vi "输入数据解析.vi"(0 "单个参数补充":dbl, 1 "从板号":dbl=1.0, 2 "主板二维码":string="BNET01", 3 "从板二维码":string="BNET01", 5 "主板引用":refnum<vi>, 7 "从板引用":refnum<vi>, 9 "主板选项":string="三级故障阀值", 11 "枚举":enum16{"主板", "从板"}(ring), 12 "快换":bool caption="快换写入") -> (4 "输出数组":dbl[][](array[numeric]), 6 "数组长度":dbl[](array[numeric]), 8 "循环次数":i32, 10 "命令":u32, 14 "名称":string[](array[string]), 15 "命令序号":u32[](array[numeric]))   [LabVIEW 2013] (continued)
                  disable-tunnel: w4127 -> [w4132 _]
                  frame Disabled {
                    n1628 = Unbundle By Name(w4132) -> ("充电电流过高"=w4131:dbl)
                    n1629 = call "输入分辨率计算-EV05.vi"("1字节?"=FALSE, "数值"=w4131, "偏移量"=-3000.0, "分辨率"=0.1) -> ("低字节"=w4133:dbl, "高字节1"=w4135:dbl)  [unwired: 1 in, 5 out]
                  }
                  frame Enabled {
                    w4138 = 255 ("高字节1")
                  }
                }
                n1630 = Build Array(w4130, w4128) -> (w4129:i32[])
              }
              frame 10 {
                # "放电电流过高"
                n1631 = disable-structure shown="启用" {
                  disable-tunnel: [w4147 w4150] -> w4142
                  disable-tunnel: [w4145 w4150] -> w4140
                  disable-tunnel: w4139 -> [w4144 _]
                  frame Disabled {
                    n1632 = Unbundle By Name(w4144) -> ("放电电流过高"=w4143:dbl)
                    n1633 = call "输入分辨率计算-EV05.vi"("1字节?"=FALSE, "数值"=w4143, "偏移量"=-3000.0, "分辨率"=0.1) -> ("低字节"=w4145:dbl, "高字节1"=w4147:dbl)  [unwired: 1 in, 5 out]
                  }
                  frame Enabled {
                    w4150 = 255 ("高字节1")
                  }
                }
                n1634 = Build Array(w4142, w4140) -> (w4141:i32[])
              }
              frame 11 {
                # "单组温度不均衡"
                n1635 = disable-structure shown="启用" {
                  disable-tunnel: [w4157 255 ("高字节1")] -> w4153
                  disable-tunnel: w4151 -> [w4155 _]
                  frame Disabled {
                    n1636 = Unbundle By Name(w4155) -> ("单组温度不均衡"=w4154:dbl)
                    n1637 = call "输入分辨率计算-EV05.vi"("1字节?"=TRUE, "数值"=w4154, "偏移量"=0.0, "分辨率"=1.0) -> ("高字节1"=w4157:dbl)  [unwired: 1 in, 6 out]
                  }
                  frame Enabled {
                  }
                }
                n1638 = Build Array(w4153) -> (w4152:i32[])
              }
              frame 12 {
                # "SOC过高"
                n1639 = Unbundle By Name(w4165) -> ("SOC过高"=w4164:dbl)
                n1640 = call "输入分辨率计算-EV05.vi"("1字节?"=FALSE, "数值"=w4164, "偏移量"=0.0, "分辨率"=0.1) -> ("低字节"=w4166:dbl, "高字节1"=w4167:dbl)  [unwired: 1 in, 5 out]
                n1641 = call "二进制解析-8.6.vi"("索引"=4, "数值"=w4167) -> ("低位子数组"=w4170:i32[])  [unwired: 3 out]
                n1642 = call "二进制解析-8.6.vi"("索引"=4, "数值"=w4166) -> ("低位子数组"=w4162:i32[], "高位子数组"=w4169:i32[])  [unwired: 2 out]
                n1643 = Insert Into Array(array=w4170, new element=w4169) -> (w4168:i32[])  [unwired: 1 in]
                n1644 = call "数值二进制转十进制-8.6.vi"("子数组"=w4168) -> ("十进制数值"=w4163:i32)  [unwired: 4 out]
                n1645 = disable-structure shown="启用" {
                  disable-tunnel: w4163 -> [w4178 _]
                  disable-tunnel: [w4178 255 ("高字节1")] -> w4161
                  disable-tunnel: [w4177 i32[] [] ("低位子数组 22")] -> _
                  disable-tunnel: w4162 -> [w4177 _]
                  frame Disabled {
                  }
                  frame Enabled {
                  }
                }
                n1646 = Build Array(w4161, w4161) -> (w4174:i32[])
              }
              frame 13 {
                # "SOC过低"
                n1647 = Unbundle By Name(w4187) -> ("SOC过低"=w4186:dbl)
                n1648 = call "输入分辨率计算-EV05.vi"("1字节?"=FALSE, "数值"=w4186, "偏移量"=0.0, "分辨率"=0.1) -> ("低字节"=w4184:dbl, "高字节1"=w4185:dbl)  [unwired: 1 in, 5 out]
                n1649 = call "二进制解析-8.6.vi"("索引"=4, "数值"=w4185) -> ("低位子数组"=w4182:i32[])  [unwired: 3 out]
                n1650 = disable-structure shown="启用" {
                  disable-tunnel: w4184 -> [w4194 _]
                  disable-tunnel: [w4194 255 ("高字节1")] -> w4183
                  disable-tunnel: w4182 -> [w4193 _]
                  disable-tunnel: [_ 255 ("高字节1")] -> w4181
                  frame Disabled {
                    (unwired) i32[] [] ("低位子数组 4")
                  }
                  frame Enabled {
                  }
                }
                n1651 = Build Array(w4181, w4183) -> (w4190:i32[])
              }
              frame 14 {
                # "内阻过大"
                n1652 = disable-structure shown="启用" {
                  disable-tunnel: w4199 -> [w4204 _]
                  disable-tunnel: [w4200 255 ("高字节1")] -> w4197
                  frame Disabled {
                    n1653 = Unbundle By Name(w4204) -> ("内阻过大"=w4203:dbl)
                    n1654 = call "输入分辨率计算-EV05.vi"("1字节?"=TRUE, "数值"=w4203, "分辨率"=0.1) -> ("高字节1"=w4200:dbl)  [unwired: 2 in, 6 out]
                  }
                  frame Enabled {
                  }
                }
                n1655 = Build Array(w4197) -> (w4198:i32[])
              }
              frame 15 {
                # "极柱温度过高"
                n1656 = disable-structure shown="启用" {
                  disable-tunnel: w4208 -> [w4214 _]
                  disable-tunnel: [w4210 255 ("高字节1")] -> w4206
                  frame Disabled {
                    n1657 = Unbundle By Name(w4214) -> ("极柱温度过高"=w4213:dbl)
                    n1658 = call "输入分辨率计算-EV05.vi"("1字节?"=TRUE, "数值"=w4213, "偏移量"=-40.0, "分辨率"=1.0) -> ("高字节1"=w4210:dbl)  [unwired: 1 in, 6 out]
                  }
                  frame Enabled {
                  }
                }
                n1659 = Build Array(w4206) -> (w4207:i32[])
              }
              frame 16 {
                # "SOH过低"
                n1660 = disable-structure shown="启用" {
                  disable-tunnel: [w4231 w4239] -> w4218
                  disable-tunnel: w4217 -> [w4228 _]
                  disable-tunnel: [w4220 w4239] -> w4216
                  frame Disabled {
                    n1661 = Unbundle By Name(w4228) -> ("SOH过低"=w4227:dbl)
                    n1662 = call "输入分辨率计算-EV05.vi"("1字节?"=FALSE, "数值"=w4227, "偏移量"=0.0, "分辨率"=0.1) -> ("低字节"=w4229:dbl, "高字节1"=w4230:dbl)  [unwired: 1 in, 5 out]
                    n1663 = call "二进制解析-8.6.vi"("索引"=4, "数值"=w4230) -> ("低位子数组"=w4233:i32[])  [unwired: 3 out]
                    n1664 = call "二进制解析-8.6.vi"("索引"=4, "数值"=w4229) -> ("低位子数组"=w4222:i32[], "高位子数组"=w4232:i32[])  [unwired: 2 out]
                    n1665 = call "二进制解析-8.6.vi"("索引"=4, "数值"=0) -> ("低位子数组"=w4223:i32[])  [unwired: 3 out]
                    n1666 = Insert Into Array(array=w4233, new element=w4232) -> (w4226:i32[])  [unwired: 1 in]
                    n1667 = Insert Into Array(array=w4222, new element=w4223) -> (w4221:i32[])  [unwired: 1 in]
                    n1668 = call "数值二进制转十进制-8.6.vi"("子数组"=w4226) -> ("十进制数值"=w4231:i32)  [unwired: 4 out]
                    n1669 = call "数值二进制转十进制-8.6.vi"("子数组"=w4221) -> ("十进制数值"=w4220:i32)  [unwired: 4 out]
                  }
                  frame Enabled {
                    w4239 = 255 ("高字节1")
                  }
                }
                n1670 = Build Array(w4218, w4216) -> (w4219:i32[])
              }
            }
            n1671 = Insert Into Array(array=w4024, new element=w4025) -> (w4023:dbl[])  [unwired: 1 in]
          }
          n1672 = Build Array(w4020) -> (w4019:dbl[][])
          n1673 = Build Array("二级故障阀值") -> (w4010:string[])
        }
        frame "整组温度不均衡(3)" {
          n1674 = Unbundle By Name(w4245) -> ("一级故障 3"=w4246:refnum<vi>)
          n1675 = property class="Clust (严格)"(reference=w4246) -> ("Value"=w4244:T4)  [unwired: 1 in, 2 out]
          n1676 = for {
            N: 17 -> [_]
            tunnel: w4244 -> [w4256]
            shift-right: [w4253] -> w4250
            shift-left: dbl[] [] -> [w4254]
            i -> [w4257]
            n1677 = case shown="4" w4257 {
              tunnel: w4256 -> [w4258 w4269 w4280 w4290 w4300 w4309 w4321 w4333 w4345 w4357 w4369 w4381 w4395 w4417 w4429 w4438 w4447]
              tunnel: [w4259 w4270 w4281 w4291 w4301 w4311 w4323 w4335 w4347 w4359 w4371 w4382 w4404 w4420 w4428 w4437 w4449] -> w4255
              frame 0, Default {
                # "总电压过高"
                n1678 = disable-structure shown="启用" {
                  disable-tunnel: [w4265 w4268] -> w4261
                  disable-tunnel: [w4264 w4268] -> w4260
                  disable-tunnel: w4258 -> [w4263 _]
                  frame Disabled {
                    n1679 = Unbundle By Name(w4263) -> ("总电压过高"=w4262:dbl)
                    n1680 = call "输入分辨率计算-EV05.vi"("1字节?"=FALSE, "数值"=w4262, "分辨率"=0.1) -> ("低字节"=w4265:dbl, "高字节1"=w4264:dbl)  [unwired: 2 in, 5 out]
                  }
                  frame Enabled {
                    w4268 = 255 ("高字节1")
                  }
                }
                n1681 = Build Array(w4260, w4261) -> (w4259:i32[])
              }
              frame 1 {
                # "总电压过低"
                n1682 = disable-structure shown="启用" {
                  disable-tunnel: [w4276 w4279] -> w4272
                  disable-tunnel: [w4275 w4279] -> w4271
                  disable-tunnel: w4269 -> [w4274 _]
                  frame Disabled {
                    n1683 = Unbundle By Name(w4274) -> ("总电压过低"=w4273:dbl)
                    n1684 = call "输入分辨率计算-EV05.vi"("1字节?"=FALSE, "数值"=w4273, "分辨率"=0.1) -> ("低字节"=w4276:dbl, "高字节1"=w4275:dbl)  [unwired: 2 in, 5 out]
                  }
                  frame Enabled {
                    w4279 = 255 ("高字节1")
                  }
                }
                n1685 = Build Array(w4271, w4272) -> (w4270:i32[])
              }
              frame 2 {
                # "温度过高"
                n1686 = disable-structure shown="启用" {
                  disable-tunnel: [w4286 255 ("高字节1")] -> w4282
                  disable-tunnel: w4280 -> [w4284 _]
                  frame Disabled {
                    n1687 = Unbundle By Name(w4284) -> ("温度过高"=w4283:dbl)
                    n1688 = call "输入分辨率计算-EV05.vi"("1字节?"=TRUE, "数值"=w4283, "偏移量"=-40.0, "分辨率"=1.0) -> ("高字节1"=w4286:dbl)  [unwired: 1 in, 6 out]
                  }
                  frame Enabled {
                  }
                }
                n1689 = Build Array(w4282) -> (w4281:i32[])
              }
              frame 3 {
                # "温度过低"
                n1690 = disable-structure shown="启用" {
                  disable-tunnel: [w4296 255 ("高字节1")] -> w4292
                  disable-tunnel: w4290 -> [w4294 _]
                  frame Disabled {
                    n1691 = Unbundle By Name(w4294) -> ("温度过低"=w4293:dbl)
                    n1692 = call "输入分辨率计算-EV05.vi"("1字节?"=TRUE, "数值"=w4293, "偏移量"=-40.0, "分辨率"=1.0) -> ("高字节1"=w4296:dbl)  [unwired: 1 in, 6 out]
                  }
                  frame Enabled {
                  }
                }
                n1693 = Build Array(w4292) -> (w4291:i32[])
              }
              frame 4 {
                # "整组温度不均衡"
                n1694 = disable-structure shown="启用" {
                  disable-tunnel: [w4305 255 ("高字节1")] -> w4302
                  disable-tunnel: w4300 -> [w4304 _]
                  frame Enabled {
                    n1695 = Unbundle By Name(w4304) -> ("整组温度不均衡"=w4303:dbl)
                    n1696 = call "输入分辨率计算-EV05.vi"("1字节?"=TRUE, "数值"=w4303, "分辨率"=1.0) -> ("高字节1"=w4305:dbl)  [unwired: 2 in, 6 out]
                  }
                  frame Disabled {
                  }
                }
                n1697 = Build Array(w4302) -> (w4301:dbl[])
              }
              frame 5 {
                # "单组电压不均衡"
                n1698 = disable-structure shown="启用" {
                  disable-tunnel: [w4317 w4320] -> w4312
                  disable-tunnel: [w4315 w4320] -> w4310
                  disable-tunnel: w4309 -> [w4314 _]
                  frame Disabled {
                    n1699 = Unbundle By Name(w4314) -> ("单组电压不均衡"=w4313:dbl)
                    n1700 = call "输入分辨率计算-EV05.vi"("1字节?"=FALSE, "数值"=w4313, "偏移量"=0.0, "分辨率"=0.001) -> ("低字节"=w4315:dbl, "高字节1"=w4317:dbl)  [unwired: 1 in, 5 out]
                  }
                  frame Enabled {
                    w4320 = 255 ("高字节1")
                  }
                }
                n1701 = Build Array(w4312, w4310) -> (w4311:i32[])
              }
              frame 6 {
                # "整组电压不均衡"
                n1702 = disable-structure shown="启用" {
                  disable-tunnel: [w4329 w4332] -> w4324
                  disable-tunnel: [w4327 w4332] -> w4322
                  disable-tunnel: w4321 -> [w4326 _]
                  frame Disabled {
                    n1703 = Unbundle By Name(w4326) -> ("整组电压不均衡"=w4325:dbl)
                    n1704 = call "输入分辨率计算-EV05.vi"("1字节?"=FALSE, "数值"=w4325, "偏移量"=0.0, "分辨率"=0.001) -> ("低字节"=w4327:dbl, "高字节1"=w4329:dbl)  [unwired: 1 in, 5 out]
                  }
                  frame Enabled {
                    w4332 = 255 ("高字节1")
                  }
                }
                n1705 = Build Array(w4324, w4322) -> (w4323:i32[])
              }
              frame 7 {
                # "单体电压过高"
                n1706 = disable-structure shown="启用" {
                  disable-tunnel: [w4341 w4344] -> w4336
                  disable-tunnel: [w4339 w4344] -> w4334
                  disable-tunnel: w4333 -> [w4338 _]
                  frame Disabled {
                    n1707 = Unbundle By Name(w4338) -> ("单体电压过高"=w4337:dbl)
                    n1708 = call "输入分辨率计算-EV05.vi"("1字节?"=FALSE, "数值"=w4337, "偏移量"=0.0, "分辨率"=0.001) -> ("低字节"=w4339:dbl, "高字节1"=w4341:dbl)  [unwired: 1 in, 5 out]
                  }
                  frame Enabled {
                    w4344 = 255 ("高字节1")
                  }
                }
                n1709 = Build Array(w4336, w4334) -> (w4335:i32[])
              }
              frame 8 {
                # "单体电压过低"
                n1710 = disable-structure shown="启用" {
                  disable-tunnel: [w4353 w4356] -> w4348
                  disable-tunnel: [w4351 w4356] -> w4346
                  disable-tunnel: w4345 -> [w4350 _]
                  frame Disabled {
                    n1711 = Unbundle By Name(w4350) -> ("单体电压过低"=w4349:dbl)
                    n1712 = call "输入分辨率计算-EV05.vi"("1字节?"=FALSE, "数值"=w4349, "偏移量"=0.0, "分辨率"=0.001) -> ("低字节"=w4351:dbl, "高字节1"=w4353:dbl)  [unwired: 1 in, 5 out]
                  }
                  frame Enabled {
                    w4356 = 255 ("高字节1")
                  }
                }
                n1713 = Build Array(w4348, w4346) -> (w4347:i32[])
              }
              frame 9 {
                # "充电电流过高"
                n1714 = disable-structure shown="启用" {
                  disable-tunnel: [w4365 w4368] -> w4360
                  disable-tunnel: [w4363 w4368] -> w4358
                  disable-tunnel: w4357 -> [w4362 _]
                  frame Disabled {
                    n1715 = Unbundle By Name(w4362) -> ("充电电流过高"=w4361:dbl)
                    n1716 = call "输入分辨率计算-EV05.vi"("1字节?"=FALSE, "数值"=w4361, "偏移量"=-3000.0, "分辨率"=0.1) -> ("低字节"=w4363:dbl, "高字节1"=w4365:dbl)  [unwired: 1 in, 5 out]
                  }
                  frame Enabled {
                    w4368 = 255 ("高字节1")
                  }
                }
                n1717 = Build Array(w4360, w4358) -> (w4359:i32[])
              }
              frame 10 {
                # "放电电流过高"
                n1718 = disable-structure shown="启用" {
                  disable-tunnel: [w4377 w4380] -> w4372
                  disable-tunnel: [w4375 w4380] -> w4370
                  disable-tunnel: w4369 -> [w4374 _]
                  frame Disabled {
                    n1719 = Unbundle By Name(w4374) -> ("放电电流过高"=w4373:dbl)
                    n1720 = call "输入分辨率计算-EV05.vi"("1字节?"=FALSE, "数值"=w4373, "偏移量"=-3000.0, "分辨率"=0.1) -> ("低字节"=w4375:dbl, "高字节1"=w4377:dbl)  [unwired: 1 in, 5 out]
                  }
                  frame Enabled {
                    w4380 = 255 ("高字节1")
                  }
                }
                n1721 = Build Array(w4372, w4370) -> (w4371:i32[])
              }
              frame 11 {
                # "单组温度不均衡"
                n1722 = disable-structure shown="启用" {
                  disable-tunnel: [w4387 255 ("高字节1")] -> w4383
                  disable-tunnel: w4381 -> [w4385 _]
                  frame Disabled {
                    n1723 = Unbundle By Name(w4385) -> ("单组温度不均衡"=w4384:dbl)
                    n1724 = call "输入分辨率计算-EV05.vi"("1字节?"=TRUE, "数值"=w4384, "偏移量"=0.0, "分辨率"=1.0) -> ("高字节1"=w4387:dbl)  [unwired: 1 in, 6 out]
                  }
                  frame Enabled {
                  }
                }
                n1725 = Build Array(w4383) -> (w4382:i32[])
              }
              frame 12 {
                # "SOC过高"
                n1726 = Unbundle By Name(w4395) -> ("SOC过高"=w4394:dbl)
                n1727 = call "输入分辨率计算-EV05.vi"("1字节?"=FALSE, "数值"=w4394, "偏移量"=0.0, "分辨率"=0.1) -> ("低字节"=w4396:dbl, "高字节1"=w4397:dbl)  [unwired: 1 in, 5 out]
                n1728 = call "二进制解析-8.6.vi"("索引"=4, "数值"=w4397) -> ("低位子数组"=w4400:i32[])  [unwired: 3 out]
                n1729 = call "二进制解析-8.6.vi"("索引"=4, "数值"=w4396) -> ("低位子数组"=w4392:i32[], "高位子数组"=w4399:i32[])  [unwired: 2 out]
                n1730 = Insert Into Array(array=w4400, new element=w4399) -> (w4398:i32[])  [unwired: 1 in]
                n1731 = call "数值二进制转十进制-8.6.vi"("子数组"=w4398) -> ("十进制数值"=w4393:i32)  [unwired: 4 out]
                n1732 = disable-structure shown="启用" {
                  disable-tunnel: w4393 -> [w4408 _]
                  disable-tunnel: [w4408 255 ("高字节1")] -> w4391
                  disable-tunnel: [w4407 i32[] [] ("低位子数组 22")] -> _
                  disable-tunnel: w4392 -> [w4407 _]
                  frame Disabled {
                  }
                  frame Enabled {
                  }
                }
                n1733 = Build Array(w4391, w4391) -> (w4404:i32[])
              }
              frame 13 {
                # "SOC过低"
                n1734 = Unbundle By Name(w4417) -> ("SOC过低"=w4416:dbl)
                n1735 = call "输入分辨率计算-EV05.vi"("1字节?"=FALSE, "数值"=w4416, "偏移量"=0.0, "分辨率"=0.1) -> ("低字节"=w4414:dbl, "高字节1"=w4415:dbl)  [unwired: 1 in, 5 out]
                n1736 = call "二进制解析-8.6.vi"("索引"=4, "数值"=w4415) -> ("低位子数组"=w4412:i32[])  [unwired: 3 out]
                n1737 = disable-structure shown="启用" {
                  disable-tunnel: w4414 -> [w4424 _]
                  disable-tunnel: [w4424 255 ("高字节1")] -> w4413
                  disable-tunnel: w4412 -> [w4423 _]
                  disable-tunnel: [_ 255 ("高字节1")] -> w4411
                  frame Disabled {
                    (unwired) i32[] [] ("低位子数组 4")
                  }
                  frame Enabled {
                  }
                }
                n1738 = Build Array(w4411, w4413) -> (w4420:i32[])
              }
              frame 14 {
                # "内阻过大"
                n1739 = disable-structure shown="启用" {
                  disable-tunnel: w4429 -> [w4434 _]
                  disable-tunnel: [w4430 255 ("高字节1")] -> w4427
                  frame Disabled {
                    n1740 = Unbundle By Name(w4434) -> ("内阻过大"=w4433:dbl)
                    n1741 = call "输入分辨率计算-EV05.vi"("1字节?"=TRUE, "数值"=w4433, "分辨率"=0.1) -> ("高字节1"=w4430:dbl)  [unwired: 2 in, 6 out]
                  }
                  frame Enabled {
                  }
                }
                n1742 = Build Array(w4427) -> (w4428:i32[])
              }
              frame 15 {
                # "极柱温度过高"
                n1743 = disable-structure shown="启用" {
                  disable-tunnel: w4438 -> [w4444 _]
                  disable-tunnel: [w4440 255 ("高字节1")] -> w4436
                  frame Disabled {
                    n1744 = Unbundle By Name(w4444) -> ("极柱温度过高"=w4443:dbl)
                    n1745 = call "输入分辨率计算-EV05.vi"("1字节?"=TRUE, "数值"=w4443, "偏移量"=-40.0, "分辨率"=1.0) -> ("高字节1"=w4440:dbl)  [unwired: 1 in, 6 out]
                  }
                  frame Enabled {
                  }
                }
                n1746 = Build Array(w4436) -> (w4437:i32[])
              }
              frame 16 {
                # "SOH过低"
                n1747 = disable-structure shown="启用" {
                  disable-tunnel: [w4461 w4469] -> w4448
                  disable-tunnel: w4447 -> [w4458 _]
                  disable-tunnel: [w4450 w4469] -> w4446
                  frame Disabled {
                    n1748 = Unbundle By Name(w4458) -> ("SOH过低"=w4457:dbl)
                    n1749 = call "输入分辨率计算-EV05.vi"("1字节?"=FALSE, "数值"=w4457, "偏移量"=0.0, "分辨率"=0.1) -> ("低字节"=w4459:dbl, "高字节1"=w4460:dbl)  [unwired: 1 in, 5 out]
                    n1750 = call "二进制解析-8.6.vi"("索引"=4, "数值"=w4460) -> ("低位子数组"=w4463:i32[])  [unwired: 3 out]
                    n1751 = call "二进制解析-8.6.vi"("索引"=4, "数值"=w4459) -> ("低位子数组"=w4452:i32[], "高位子数组"=w4462:i32[])  [unwired: 2 out]
                    n1752 = call "二进制解析-8.6.vi"("索引"=4, "数值"=0) -> ("低位子数组"=w4453:i32[])  [unwired: 3 out]
                    n1753 = Insert Into Array(array=w4463, new element=w4462) -> (w4456:i32[])  [unwired: 1 in]
                    n1754 = Insert Into Array(array=w4452, new element=w4453) -> (w4451:i32[])  [unwired: 1 in]
                    n1755 = call "数值二进制转十进制-8.6.vi"("子数组"=w4456) -> ("十进制数值"=w4461:i32)  [unwired: 4 out]
                    n1756 = call "数值二进制转十进制-8.6.vi"("子数组"=w4451) -> ("十进制数值"=w4450:i32)  [unwired: 4 out]
                  }
                  frame Enabled {
                    w4469 = 255 ("高字节1")
                  }
                }
                n1757 = Build Array(w4448, w4446) -> (w4449:i32[])
              }
            }
            n1758 = Insert Into Array(array=w4254, new element=w4255) -> (w4253:dbl[])  [unwired: 1 in]
          }
          n1759 = Build Array(w4250) -> (w4249:dbl[][])
          n1760 = Build Array("三级故障阀值") -> (w4240:string[])
        }
        frame "单组电压不均衡" {
          n1761 = Unbundle By Name(w4475) -> ("一级故障"=w4476:refnum<vi>)
          n1762 = property class="Clust (严格)"(reference=w4476) -> ("Value"=w4474:T4)  [unwired: 1 in, 2 out]
          n1763 = for {
            N: 17 -> [_]
            tunnel: w4474 -> [w4486]
            shift-right: [w4483] -> w4480
            shift-left: dbl[] [] -> [w4484]
            i -> [w4487]
            n1764 = case shown="13" w4487 {
              tunnel: w4486 -> [w4488 w4499 w4510 w4520 w4530 w4540 w4552 w4564 w4576 w4588 w4600 w4612 w4626 w4648 w4660 w4669 w4678]
              tunnel: [w4489 w4500 w4511 w4521 w4531 w4542 w4554 w4566 w4578 w4590 w4602 w4613 w4635 w4651 w4659 w4668 w4680] -> w4485
              frame 0, Default {
                # "总电压过高"
                n1765 = disable-structure shown="启用" {
                  disable-tunnel: [w4495 w4498] -> w4491
                  disable-tunnel: [w4494 w4498] -> w4490
                  disable-tunnel: w4488 -> [w4493 _]
                  frame Disabled {
                    n1766 = Unbundle By Name(w4493) -> ("总电压过高"=w4492:dbl)
                    n1767 = call "输入分辨率计算-EV05.vi"("1字节?"=FALSE, "数值"=w4492, "分辨率"=0.1) -> ("低字节"=w4495:dbl, "高字节1"=w4494:dbl)  [unwired: 2 in, 5 out]
                  }
                  frame Enabled {
                    w4498 = 255 ("高字节1")
                  }
                }
                n1768 = Build Array(w4490, w4491) -> (w4489:i32[])
              }
              frame 1 {
                # "总电压过低"
                n1769 = disable-structure shown="启用" {
                  disable-tunnel: [w4506 w4509] -> w4502
                  disable-tunnel: [w4505 w4509] -> w4501
                  disable-tunnel: w4499 -> [w4504 _]
                  frame Disabled {
                    n1770 = Unbundle By Name(w4504) -> ("总电压过低"=w4503:dbl)
                    n1771 = call "输入分辨率计算-EV05.vi"("1字节?"=FALSE, "数值"=w4503, "分辨率"=0.1) -> ("低字节"=w4506:dbl, "高字节1"=w4505:dbl)  [unwired: 2 in, 5 out]
                  }
                  frame Enabled {
                    w4509 = 255 ("高字节1")
                  }
                }
                n1772 = Build Array(w4501, w4502) -> (w4500:i32[])
              }
              frame 2 {
                # "温度过高"
                n1773 = disable-structure shown="启用" {
                  disable-tunnel: [w4516 255 ("高字节1")] -> w4512
                  disable-tunnel: w4510 -> [w4514 _]
                  frame Disabled {
                    n1774 = Unbundle By Name(w4514) -> ("温度过高"=w4513:dbl)
                    n1775 = call "输入分辨率计算-EV05.vi"("1字节?"=TRUE, "数值"=w4513, "偏移量"=-40.0, "分辨率"=1.0) -> ("高字节1"=w4516:dbl)  [unwired: 1 in, 6 out]
                  }
                  frame Enabled {
                  }
                }
                n1776 = Build Array(w4512) -> (w4511:i32[])
              }
              frame 3 {
                # "温度过低"
                n1777 = disable-structure shown="启用" {
                  disable-tunnel: [w4526 255 ("高字节1")] -> w4522
                  disable-tunnel: w4520 -> [w4524 _]
                  frame Disabled {
                    n1778 = Unbundle By Name(w4524) -> ("温度过低"=w4523:dbl)
                    n1779 = call "输入分辨率计算-EV05.vi"("1字节?"=TRUE, "数值"=w4523, "偏移量"=-40.0, "分辨率"=1.0) -> ("高字节1"=w4526:dbl)  [unwired: 1 in, 6 out]
                  }
                  frame Enabled {
                  }
                }
                n1780 = Build Array(w4522) -> (w4521:i32[])
              }
              frame 4 {
                # "整组温度不均衡"
                n1781 = disable-structure shown="启用" {
                  disable-tunnel: [w4536 255 ("高字节1")] -> w4532
                  disable-tunnel: w4530 -> [w4534 _]
                  frame Disabled {
                    n1782 = Unbundle By Name(w4534) -> ("整组温度不均衡"=w4533:dbl)
                    n1783 = call "输入分辨率计算-EV05.vi"("1字节?"=TRUE, "数值"=w4533, "偏移量"=0.0, "分辨率"=1.0) -> ("高字节1"=w4536:dbl)  [unwired: 1 in, 6 out]
                  }
                  frame Enabled {
                  }
                }
                n1784 = Build Array(w4532) -> (w4531:i32[])
              }
              frame 5 {
                # "单组电压不均衡"
                n1785 = disable-structure shown="启用" {
                  disable-tunnel: [w4548 w4551] -> w4543
                  disable-tunnel: [w4546 w4551] -> w4541
                  disable-tunnel: w4540 -> [w4545 _]
                  frame Enabled {
                    n1786 = Unbundle By Name(w4545) -> ("单组电压不均衡"=w4544:dbl)
                    n1787 = call "输入分辨率计算-EV05.vi"("1字节?"=FALSE, "数值"=w4544, "偏移量"=0.0, "分辨率"=0.001) -> ("低字节"=w4546:dbl, "高字节1"=w4548:dbl)  [unwired: 1 in, 5 out]
                  }
                  frame Disabled {
                    w4551 = 255 ("高字节1")
                  }
                }
                n1788 = Build Array(w4543, w4541) -> (w4542:dbl[])
              }
              frame 6 {
                # "整组电压不均衡"
                n1789 = disable-structure shown="启用" {
                  disable-tunnel: [w4560 w4563] -> w4555
                  disable-tunnel: [w4558 w4563] -> w4553
                  disable-tunnel: w4552 -> [w4557 _]
                  frame Disabled {
                    n1790 = Unbundle By Name(w4557) -> ("整组电压不均衡"=w4556:dbl)
                    n1791 = call "输入分辨率计算-EV05.vi"("1字节?"=FALSE, "数值"=w4556, "偏移量"=0.0, "分辨率"=0.001) -> ("低字节"=w4558:dbl, "高字节1"=w4560:dbl)  [unwired: 1 in, 5 out]
                  }
                  frame Enabled {
                    w4563 = 255 ("高字节1")
                  }
                }
                n1792 = Build Array(w4555, w4553) -> (w4554:i32[])
              }
              frame 7 {
                # "单体电压过高"
                n1793 = disable-structure shown="启用" {
                  disable-tunnel: [w4572 w4575] -> w4567
                  disable-tunnel: [w4570 w4575] -> w4565
                  disable-tunnel: w4564 -> [w4569 _]
                  frame Disabled {
                    n1794 = Unbundle By Name(w4569) -> ("单体电压过高"=w4568:dbl)
                    n1795 = call "输入分辨率计算-EV05.vi"("1字节?"=FALSE, "数值"=w4568, "偏移量"=0.0, "分辨率"=0.001) -> ("低字节"=w4570:dbl, "高字节1"=w4572:dbl)  [unwired: 1 in, 5 out]
                  }
                  frame Enabled {
                    w4575 = 255 ("高字节1")
                  }
                }
                n1796 = Build Array(w4567, w4565) -> (w4566:i32[])
              }
              frame 8 {
                # "单体电压过低"
                n1797 = disable-structure shown="启用" {
                  disable-tunnel: [w4584 w4587] -> w4579
                  disable-tunnel: [w4582 w4587] -> w4577
                  disable-tunnel: w4576 -> [w4581 _]
                  frame Disabled {
                    n1798 = Unbundle By Name(w4581) -> ("单体电压过低"=w4580:dbl)
                    n1799 = call "输入分辨率计算-EV05.vi"("1字节?"=FALSE, "数值"=w4580, "偏移量"=0.0, "分辨率"=0.001) -> ("低字节"=w4582:dbl, "高字节1"=w4584:dbl)  [unwired: 1 in, 5 out]
                  }
                  frame Enabled {
                    w4587 = 255 ("高字节1")
                  }
                }
                n1800 = Build Array(w4579, w4577) -> (w4578:i32[])
              }
              frame 9 {
                # "充电电流过高"
                n1801 = disable-structure shown="启用" {
                  disable-tunnel: [w4596 w4599] -> w4591
                  disable-tunnel: [w4594 w4599] -> w4589
                  disable-tunnel: w4588 -> [w4593 _]
                  frame Disabled {
                    n1802 = Unbundle By Name(w4593) -> ("充电电流过高"=w4592:dbl)
                    n1803 = call "输入分辨率计算-EV05.vi"("1字节?"=FALSE, "数值"=w4592, "偏移量"=-3000.0, "分辨率"=0.1) -> ("低字节"=w4594:dbl, "高字节1"=w4596:dbl)  [unwired: 1 in, 5 out]
                  }
                  frame Enabled {
                    w4599 = 255 ("高字节1")
                  }
                }
                n1804 = Build Array(w4591, w4589) -> (w4590:i32[])
              }
              frame 10 {
                # "放电电流过高"
                n1805 = disable-structure shown="启用" {
                  disable-tunnel: [w4608 w4611] -> w4603
                  disable-tunnel: [w4606 w4611] -> w4601
                  disable-tunnel: w4600 -> [w4605 _]
                  frame Disabled {
                    n1806 = Unbundle By Name(w4605) -> ("放电电流过高"=w4604:dbl)
                    n1807 = call "输入分辨率计算-EV05.vi"("1字节?"=FALSE, "数值"=w4604, "偏移量"=-3000.0, "分辨率"=0.1) -> ("低字节"=w4606:dbl, "高字节1"=w4608:dbl)  [unwired: 1 in, 5 out]
                  }
                  frame Enabled {
                    w4611 = 255 ("高字节1")
                  }
                }
                n1808 = Build Array(w4603, w4601) -> (w4602:i32[])
              }
              frame 11 {
                # "单组温度不均衡"
                n1809 = disable-structure shown="启用" {
                  disable-tunnel: [w4618 255 ("高字节1")] -> w4614
                  disable-tunnel: w4612 -> [w4616 _]
                  frame Disabled {
                    n1810 = Unbundle By Name(w4616) -> ("单组温度不均衡"=w4615:dbl)
                    n1811 = call "输入分辨率计算-EV05.vi"("1字节?"=TRUE, "数值"=w4615, "偏移量"=0.0, "分辨率"=1.0) -> ("高字节1"=w4618:dbl)  [unwired: 1 in, 6 out]
                  }
                  frame Enabled {
                  }
                }
                n1812 = Build Array(w4614) -> (w4613:i32[])
              }
              frame 12 {
                # "SOC过高"
                n1813 = Unbundle By Name(w4626) -> ("SOC过高"=w4625:dbl)
                n1814 = call "输入分辨率计算-EV05.vi"("1字节?"=FALSE, "数值"=w4625, "偏移量"=0.0, "分辨率"=0.1) -> ("低字节"=w4627:dbl, "高字节1"=w4628:dbl)  [unwired: 1 in, 5 out]
                n1815 = call "二进制解析-8.6.vi"("索引"=4, "数值"=w4628) -> ("低位子数组"=w4631:i32[])  [unwired: 3 out]
                n1816 = call "二进制解析-8.6.vi"("索引"=4, "数值"=w4627) -> ("低位子数组"=w4623:i32[], "高位子数组"=w4630:i32[])  [unwired: 2 out]
                n1817 = Insert Into Array(array=w4631, new element=w4630) -> (w4629:i32[])  [unwired: 1 in]
                n1818 = call "数值二进制转十进制-8.6.vi"("子数组"=w4629) -> ("十进制数值"=w4624:i32)  [unwired: 4 out]
                n1819 = disable-structure shown="启用" {
                  disable-tunnel: w4624 -> [w4639 _]
                  disable-tunnel: [w4639 255 ("高字节1")] -> w4622
                  disable-tunnel: [w4638 i32[] [] ("低位子数组 23")] -> _
                  disable-tunnel: w4623 -> [w4638 _]
                  frame Disabled {
                  }
                  frame Enabled {
                  }
                }
                n1820 = Build Array(w4622, w4622) -> (w4635:i32[])
              }
              frame 13 {
                # "SOC过低"
                n1821 = Unbundle By Name(w4648) -> ("SOC过低"=w4647:dbl)
                n1822 = call "输入分辨率计算-EV05.vi"("1字节?"=FALSE, "数值"=w4647, "偏移量"=0.0, "分辨率"=0.1) -> ("低字节"=w4645:dbl, "高字节1"=w4646:dbl)  [unwired: 1 in, 5 out]
                n1823 = call "二进制解析-8.6.vi"("索引"=4, "数值"=w4646) -> ("低位子数组"=w4643:i32[])  [unwired: 3 out]
                n1824 = disable-structure shown="启用" {
                  disable-tunnel: w4645 -> [w4655 _]
                  disable-tunnel: [w4655 255 ("高字节1")] -> w4644
                  disable-tunnel: w4643 -> [w4654 _]
                  disable-tunnel: [_ 255 ("高字节1")] -> w4642
                  frame Disabled {
                    (unwired) i32[] [] ("低位子数组 4")
                  }
                  frame Enabled {
                  }
                }
                n1825 = Build Array(w4642, w4644) -> (w4651:i32[])
              }
              frame 14 {
                # "内阻过大"
                n1826 = disable-structure shown="启用" {
                  disable-tunnel: w4660 -> [w4665 _]
                  disable-tunnel: [w4661 255 ("高字节1")] -> w4658
                  frame Disabled {
                    n1827 = Unbundle By Name(w4665) -> ("内阻过大"=w4664:dbl)
                    n1828 = call "输入分辨率计算-EV05.vi"("1字节?"=TRUE, "数值"=w4664, "分辨率"=0.1) -> ("高字节1"=w4661:dbl)  [unwired: 2 in, 6 out]
                  }
                  frame Enabled {
                  }
                }
                n1829 = Build Array(w4658) -> (w4659:i32[])
              }
              frame 15 {
                # "极柱温度过高"
                n1830 = disable-structure shown="启用" {
                  disable-tunnel: w4669 -> [w4675 _]
                  disable-tunnel: [w4671 255 ("高字节1")] -> w4667
                  frame Disabled {
                    n1831 = Unbundle By Name(w4675) -> ("极柱温度过高"=w4674:dbl)
                    n1832 = call "输入分辨率计算-EV05.vi"("1字节?"=TRUE, "数值"=w4674, "偏移量"=-40.0, "分辨率"=1.0) -> ("高字节1"=w4671:dbl)  [unwired: 1 in, 6 out]
                  }
                  frame Enabled {
                  }
                }
                n1833 = Build Array(w4667) -> (w4668:i32[])
              }
              frame 16 {
                # "SOH过低"
                n1834 = disable-structure shown="启用" {
                  disable-tunnel: [w4692 w4700] -> w4679
                  disable-tunnel: w4678 -> [w4689 _]
                  disable-tunnel: [w4681 w4700] -> w4677
                  frame Disabled {
                    n1835 = Unbundle By Name(w4689) -> ("SOH过低"=w4688:dbl)
                    n1836 = call "输入分辨率计算-EV05.vi"("1字节?"=FALSE, "数值"=w4688, "偏移量"=0.0, "分辨率"=0.1) -> ("低字节"=w4690:dbl, "高字节1"=w4691:dbl)  [unwired: 1 in, 5 out]
                    n1837 = call "二进制解析-8.6.vi"("索引"=4, "数值"=w4691) -> ("低位子数组"=w4694:i32[])  [unwired: 3 out]
                    n1838 = call "二进制解析-8.6.vi"("索引"=4, "数值"=w4690) -> ("低位子数组"=w4683:i32[], "高位子数组"=w4693:i32[])  [unwired: 2 out]
                    n1839 = call "二进制解析-8.6.vi"("索引"=4, "数值"=0) -> ("低位子数组"=w4684:i32[])  [unwired: 3 out]
                    n1840 = Insert Into Array(array=w4694, new element=w4693) -> (w4687:i32[])  [unwired: 1 in]
                    n1841 = Insert Into Array(array=w4683, new element=w4684) -> (w4682:i32[])  [unwired: 1 in]
                    n1842 = call "数值二进制转十进制-8.6.vi"("子数组"=w4687) -> ("十进制数值"=w4692:i32)  [unwired: 4 out]
                    n1843 = call "数值二进制转十进制-8.6.vi"("子数组"=w4682) -> ("十进制数值"=w4681:i32)  [unwired: 4 out]
                  }
                  frame Enabled {
                    w4700 = 255 ("高字节1")
                  }
                }
                n1844 = Build Array(w4679, w4677) -> (w4680:i32[])
              }
            }
            n1845 = Insert Into Array(array=w4484, new element=w4485) -> (w4483:dbl[])  [unwired: 1 in]
          }
          n1846 = Build Array(w4480) -> (w4479:dbl[][])
          n1847 = Build Array("一级故障阀值") -> (w4470:string[])
        }
        frame "单组电压不均衡(2)" {
          n1848 = Unbundle By Name(w4706) -> ("一级故障 2"=w4707:refnum<vi>)
          n1849 = property class="Clust (严格)"(reference=w4707) -> ("Value"=w4705:T4)  [unwired: 1 in, 2 out]
          n1850 = for {
            N: 17 -> [_]
            tunnel: w4705 -> [w4717]
            shift-right: [w4714] -> w4711
            shift-left: dbl[] [] -> [w4715]
            i -> [w4718]
            n1851 = case shown="13" w4718 {
              tunnel: w4717 -> [w4719 w4730 w4741 w4751 w4761 w4771 w4783 w4795 w4807 w4819 w4831 w4843 w4857 w4879 w4891 w4900 w4909]
              tunnel: [w4720 w4731 w4742 w4752 w4762 w4773 w4785 w4797 w4809 w4821 w4833 w4844 w4866 w4882 w4890 w4899 w4911] -> w4716
              frame 0, Default {
                # "总电压过高"
                n1852 = disable-structure shown="启用" {
                  disable-tunnel: [w4726 w4729] -> w4722
                  disable-tunnel: [w4725 w4729] -> w4721
                  disable-tunnel: w4719 -> [w4724 _]
                  frame Disabled {
                    n1853 = Unbundle By Name(w4724) -> ("总电压过高"=w4723:dbl)
                    n1854 = call "输入分辨率计算-EV05.vi"("1字节?"=FALSE, "数值"=w4723, "分辨率"=0.1) -> ("低字节"=w4726:dbl, "高字节1"=w4725:dbl)  [unwired: 2 in, 5 out]
                  }
                  frame Enabled {
                    w4729 = 255 ("高字节1")
                  }
                }
                n1855 = Build Array(w4721, w4722) -> (w4720:i32[])
              }
              frame 1 {
                # "总电压过低"
                n1856 = disable-structure shown="启用" {
                  disable-tunnel: [w4737 w4740] -> w4733
                  disable-tunnel: [w4736 w4740] -> w4732
                  disable-tunnel: w4730 -> [w4735 _]
                  frame Disabled {
                    n1857 = Unbundle By Name(w4735) -> ("总电压过低"=w4734:dbl)
                    n1858 = call "输入分辨率计算-EV05.vi"("1字节?"=FALSE, "数值"=w4734, "分辨率"=0.1) -> ("低字节"=w4737:dbl, "高字节1"=w4736:dbl)  [unwired: 2 in, 5 out]
                  }
                  frame Enabled {
                    w4740 = 255 ("高字节1")
                  }
                }
                n1859 = Build Array(w4732, w4733) -> (w4731:i32[])
              }
              frame 2 {
                # "温度过高"
                n1860 = disable-structure shown="启用" {
                  disable-tunnel: [w4747 255 ("高字节1")] -> w4743
                  disable-tunnel: w4741 -> [w4745 _]
                  frame Disabled {
                    n1861 = Unbundle By Name(w4745) -> ("温度过高"=w4744:dbl)
                    n1862 = call "输入分辨率计算-EV05.vi"("1字节?"=TRUE, "数值"=w4744, "偏移量"=-40.0, "分辨率"=1.0) -> ("高字节1"=w4747:dbl)  [unwired: 1 in, 6 out]
                  }
                  frame Enabled {
                  }
                }
                n1863 = Build Array(w4743) -> (w4742:i32[])
              }
              frame 3 {
                # "温度过低"
                n1864 = disable-structure shown="启用" {
                  disable-tunnel: [w4757 255 ("高字节1")] -> w4753
                  disable-tunnel: w4751 -> [w4755 _]
                  frame Disabled {
                    n1865 = Unbundle By Name(w4755) -> ("温度过低"=w4754:dbl)
                    n1866 = call "输入分辨率计算-EV05.vi"("1字节?"=TRUE, "数值"=w4754, "偏移量"=-40.0, "分辨率"=1.0) -> ("高字节1"=w4757:dbl)  [unwired: 1 in, 6 out]
                  }
                  frame Enabled {
                  }
                }
                n1867 = Build Array(w4753) -> (w4752:i32[])
              }
              frame 4 {
                # "整组温度不均衡"
                n1868 = disable-structure shown="启用" {
                  disable-tunnel: [w4767 255 ("高字节1")] -> w4763
                  disable-tunnel: w4761 -> [w4765 _]
                  frame Disabled {
                    n1869 = Unbundle By Name(w4765) -> ("整组温度不均衡"=w4764:dbl)
                    n1870 = call "输入分辨率计算-EV05.vi"("1字节?"=TRUE, "数值"=w4764, "偏移量"=0.0, "分辨率"=1.0) -> ("高字节1"=w4767:dbl)  [unwired: 1 in, 6 out]
                  }
                  frame Enabled {
                  }
                }
                n1871 = Build Array(w4763) -> (w4762:i32[])
              }
              frame 5 {
                # "单组电压不均衡"
                n1872 = disable-structure shown="启用" {
                  disable-tunnel: [w4779 w4782] -> w4774
                  disable-tunnel: [w4777 w4782] -> w4772
                  disable-tunnel: w4771 -> [w4776 _]
                  frame Enabled {
                    n1873 = Unbundle By Name(w4776) -> ("单组电压不均衡"=w4775:dbl)
                    n1874 = call "输入分辨率计算-EV05.vi"("1字节?"=FALSE, "数值"=w4775, "偏移量"=0.0, "分辨率"=0.001) -> ("低字节"=w4777:dbl, "高字节1"=w4779:dbl)  [unwired: 1 in, 5 out]
                  }
                  frame Disabled {
                    w4782 = 255 ("高字节1")
                  }
                }
                n1875 = Build Array(w4774, w4772) -> (w4773:dbl[])
              }
              frame 6 {
                # "整组电压不均衡"
                n1876 = disable-structure shown="启用" {
                  disable-tunnel: [w4791 w4794] -> w4786
                  disable-tunnel: [w4789 w4794] -> w4784
                  disable-tunnel: w4783 -> [w4788 _]
                  frame Disabled {
                    n1877 = Unbundle By Name(w4788) -> ("整组电压不均衡"=w4787:dbl)
                    n1878 = call "输入分辨率计算-EV05.vi"("1字节?"=FALSE, "数值"=w4787, "偏移量"=0.0, "分辨率"=0.001) -> ("低字节"=w4789:dbl, "高字节1"=w4791:dbl)  [unwired: 1 in, 5 out]
                  }
                  frame Enabled {
                    w4794 = 255 ("高字节1")
                  }
                }
                n1879 = Build Array(w4786, w4784) -> (w4785:i32[])
              }
              frame 7 {
                # "单体电压过高"
                n1880 = disable-structure shown="启用" {
                  disable-tunnel: [w4803 w4806] -> w4798
                  disable-tunnel: [w4801 w4806] -> w4796
                  disable-tunnel: w4795 -> [w4800 _]
                  frame Disabled {
                    n1881 = Unbundle By Name(w4800) -> ("单体电压过高"=w4799:dbl)
                    n1882 = call "输入分辨率计算-EV05.vi"("1字节?"=FALSE, "数值"=w4799, "偏移量"=0.0, "分辨率"=0.001) -> ("低字节"=w4801:dbl, "高字节1"=w4803:dbl)  [unwired: 1 in, 5 out]
                  }
                  frame Enabled {
                    w4806 = 255 ("高字节1")
                  }
                }
                n1883 = Build Array(w4798, w4796) -> (w4797:i32[])
              }
              frame 8 {
                # "单体电压过低"
                n1884 = disable-structure shown="启用" {
                  disable-tunnel: [w4815 w4818] -> w4810
                  disable-tunnel: [w4813 w4818] -> w4808
                  disable-tunnel: w4807 -> [w4812 _]
                  frame Disabled {
                    n1885 = Unbundle By Name(w4812) -> ("单体电压过低"=w4811:dbl)
                    n1886 = call "输入分辨率计算-EV05.vi"("1字节?"=FALSE, "数值"=w4811, "偏移量"=0.0, "分辨率"=0.001) -> ("低字节"=w4813:dbl, "高字节1"=w4815:dbl)  [unwired: 1 in, 5 out]
                  }
                  frame Enabled {
                    w4818 = 255 ("高字节1")
                  }
                }
                n1887 = Build Array(w4810, w4808) -> (w4809:i32[])
              }
              frame 9 {
                # "充电电流过高"
                n1888 = disable-structure shown="启用" {
                  disable-tunnel: [w4827 w4830] -> w4822
                  disable-tunnel: [w4825 w4830] -> w4820
                  disable-tunnel: w4819 -> [w4824 _]
                  frame Disabled {
                    n1889 = Unbundle By Name(w4824) -> ("充电电流过高"=w4823:dbl)
                    n1890 = call "输入分辨率计算-EV05.vi"("1字节?"=FALSE, "数值"=w4823, "偏移量"=-3000.0, "分辨率"=0.1) -> ("低字节"=w4825:dbl, "高字节1"=w4827:dbl)  [unwired: 1 in, 5 out]
                  }
                  frame Enabled {
                    w4830 = 255 ("高字节1")
                  }
                }
                n1891 = Build Array(w4822, w4820) -> (w4821:i32[])
              }
              frame 10 {
                # "放电电流过高"
                n1892 = disable-structure shown="启用" {
                  disable-tunnel: [w4839 w4842] -> w4834
                  disable-tunnel: [w4837 w4842] -> w4832
                  disable-tunnel: w4831 -> [w4836 _]
                  frame Disabled {
                    n1893 = Unbundle By Name(w4836) -> ("放电电流过高"=w4835:dbl)
                    n1894 = call "输入分辨率计算-EV05.vi"("1字节?"=FALSE, "数值"=w4835, "偏移量"=-3000.0, "分辨率"=0.1) -> ("低字节"=w4837:dbl, "高字节1"=w4839:dbl)  [unwired: 1 in, 5 out]
                  }
                  frame Enabled {
                    w4842 = 255 ("高字节1")
                  }
                }
                n1895 = Build Array(w4834, w4832) -> (w4833:i32[])
              }
              frame 11 {
                # "单组温度不均衡"
                n1896 = disable-structure shown="启用" {
                  disable-tunnel: [w4849 255 ("高字节1")] -> w4845
                  disable-tunnel: w4843 -> [w4847 _]
                  frame Disabled {
                    n1897 = Unbundle By Name(w4847) -> ("单组温度不均衡"=w4846:dbl)
                    n1898 = call "输入分辨率计算-EV05.vi"("1字节?"=TRUE, "数值"=w4846, "偏移量"=0.0, "分辨率"=1.0) -> ("高字节1"=w4849:dbl)  [unwired: 1 in, 6 out]
                  }
                  frame Enabled {
                  }
                }
                n1899 = Build Array(w4845) -> (w4844:i32[])
              }
              frame 12 {
                # "SOC过高"
                n1900 = Unbundle By Name(w4857) -> ("SOC过高"=w4856:dbl)
                n1901 = call "输入分辨率计算-EV05.vi"("1字节?"=FALSE, "数值"=w4856, "偏移量"=0.0, "分辨率"=0.1) -> ("低字节"=w4858:dbl, "高字节1"=w4859:dbl)  [unwired: 1 in, 5 out]
                n1902 = call "二进制解析-8.6.vi"("索引"=4, "数值"=w4859) -> ("低位子数组"=w4862:i32[])  [unwired: 3 out]
                n1903 = call "二进制解析-8.6.vi"("索引"=4, "数值"=w4858) -> ("低位子数组"=w4854:i32[], "高位子数组"=w4861:i32[])  [unwired: 2 out]
                n1904 = Insert Into Array(array=w4862, new element=w4861) -> (w4860:i32[])  [unwired: 1 in]
                n1905 = call "数值二进制转十进制-8.6.vi"("子数组"=w4860) -> ("十进制数值"=w4855:i32)  [unwired: 4 out]
                n1906 = disable-structure shown="启用" {
                  disable-tunnel: w4855 -> [w4870 _]
                  disable-tunnel: [w4870 255 ("高字节1")] -> w4853
                  disable-tunnel: [w4869 i32[] [] ("低位子数组 23")] -> _
                  disable-tunnel: w4854 -> [w4869 _]
                  frame Disabled {
                  }
                  frame Enabled {
                  }
                }
                n1907 = Build Array(w4853, w4853) -> (w4866:i32[])
              }
              frame 13 {
                # "SOC过低"
                n1908 = Unbundle By Name(w4879) -> ("SOC过低"=w4878:dbl)
                n1909 = call "输入分辨率计算-EV05.vi"("1字节?"=FALSE, "数值"=w4878, "偏移量"=0.0, "分辨率"=0.1) -> ("低字节"=w4876:dbl, "高字节1"=w4877:dbl)  [unwired: 1 in, 5 out]
                n1910 = call "二进制解析-8.6.vi"("索引"=4, "数值"=w4877) -> ("低位子数组"=w4874:i32[])  [unwired: 3 out]
                n1911 = disable-structure shown="启用" {
                  disable-tunnel: w4876 -> [w4886 _]
                  disable-tunnel: [w4886 255 ("高字节1")] -> w4875
                  disable-tunnel: w4874 -> [w4885 _]
                  disable-tunnel: [_ 255 ("高字节1")] -> w4873
                  frame Disabled {
                    (unwired) i32[] [] ("低位子数组 4")
                  }
                  frame Enabled {
                  }
                }
                n1912 = Build Array(w4873, w4875) -> (w4882:i32[])
              }
              frame 14 {
                # "内阻过大"
                n1913 = disable-structure shown="启用" {
                  disable-tunnel: w4891 -> [w4896 _]
                  disable-tunnel: [w4892 255 ("高字节1")] -> w4889
                  frame Disabled {
                    n1914 = Unbundle By Name(w4896) -> ("内阻过大"=w4895:dbl)
                    n1915 = call "输入分辨率计算-EV05.vi"("1字节?"=TRUE, "数值"=w4895, "分辨率"=0.1) -> ("高字节1"=w4892:dbl)  [unwired: 2 in, 6 out]
                  }
                  frame Enabled {
                  }
                }
                n1916 = Build Array(w4889) -> (w4890:i32[])
              }
              frame 15 {
                # "极柱温度过高"
                n1917 = disable-structure shown="启用" {
                  disable-tunnel: w4900 -> [w4906 _]
                  disable-tunnel: [w4902 255 ("高字节1")] -> w4898
                  frame Disabled {
                    n1918 = Unbundle By Name(w4906) -> ("极柱温度过高"=w4905:dbl)
                    n1919 = call "输入分辨率计算-EV05.vi"("1字节?"=TRUE, "数值"=w4905, "偏移量"=-40.0, "分辨率"=1.0) -> ("高字节1"=w4902:dbl)  [unwired: 1 in, 6 out]
                  }
                  frame Enabled {
                  }
                }
                n1920 = Build Array(w4898) -> (w4899:i32[])
              }
              frame 16 {
                # "SOH过低"
                n1921 = disable-structure shown="启用" {
                  disable-tunnel: [w4923 w4931] -> w4910
                  disable-tunnel: w4909 -> [w4920 _]
                  disable-tunnel: [w4912 w4931] -> w4908
                  frame Disabled {
                    n1922 = Unbundle By Name(w4920) -> ("SOH过低"=w4919:dbl)
                    n1923 = call "输入分辨率计算-EV05.vi"("1字节?"=FALSE, "数值"=w4919, "偏移量"=0.0, "分辨率"=0.1) -> ("低字节"=w4921:dbl, "高字节1"=w4922:dbl)  [unwired: 1 in, 5 out]
                    n1924 = call "二进制解析-8.6.vi"("索引"=4, "数值"=w4922) -> ("低位子数组"=w4925:i32[])  [unwired: 3 out]
                    n1925 = call "二进制解析-8.6.vi"("索引"=4, "数值"=w4921) -> ("低位子数组"=w4914:i32[], "高位子数组"=w4924:i32[])  [unwired: 2 out]
                    n1926 = call "二进制解析-8.6.vi"("索引"=4, "数值"=0) -> ("低位子数组"=w4915:i32[])  [unwired: 3 out]
                    n1927 = Insert Into Array(array=w4925, new element=w4924) -> (w4918:i32[])  [unwired: 1 in]
                    n1928 = Insert Into Array(array=w4914, new element=w4915) -> (w4913:i32[])  [unwired: 1 in]
                    n1929 = call "数值二进制转十进制-8.6.vi"("子数组"=w4918) -> ("十进制数值"=w4923:i32)  [unwired: 4 out]
                    n1930 = call "数值二进制转十进制-8.6.vi"("子数组"=w4913) -> ("十进制数值"=w4912:i32)  [unwired: 4 out]
                  }
                  frame Enabled {
                    w4931 = 255 ("高字节1")
                  }
                }
                n1931 = Build Array(w4910, w4908) -> (w4911:i32[])
              }
            }
            n1932 = Insert Into Array(array=w4715, new element=w4716) -> (w4714:dbl[])  [unwired: 1 in]
          }
          n1933 = Build Array(w4711) -> (w4710:dbl[][])
          n1934 = Build Array("二级故障阀值") -> (w4701:string[])
        }
        frame "单组电压不均衡(3)" {
          n1935 = Unbundle By Name(w4937) -> ("一级故障 3"=w4938:refnum<vi>)
          n1936 = property class="Clust (严格)"(reference=w4938) -> ("Value"=w4936:T4)  [unwired: 1 in, 2 out]
          n1937 = for {
            N: 17 -> [_]
            tunnel: w4936 -> [w4948]
            shift-right: [w4945] -> w4942
            shift-left: dbl[] [] -> [w4946]
            i -> [w4949]
            n1938 = case shown="13" w4949 {
              tunnel: w4948 -> [w4950 w4961 w4972 w4982 w4992 w5002 w5014 w5026 w5038 w5050 w5062 w5074 w5088 w5110 w5122 w5131 w5140]
              tunnel: [w4951 w4962 w4973 w4983 w4993 w5004 w5016 w5028 w5040 w5052 w5064 w5075 w5097 w5113 w5121 w5130 w5142] -> w4947
              frame 0, Default {
                # "总电压过高"
                n1939 = disable-structure shown="启用" {
                  disable-tunnel: [w4957 w4960] -> w4953
                  disable-tunnel: [w4956 w4960] -> w4952
                  disable-tunnel: w4950 -> [w4955 _]
                  frame Disabled {
                    n1940 = Unbundle By Name(w4955) -> ("总电压过高"=w4954:dbl)
                    n1941 = call "输入分辨率计算-EV05.vi"("1字节?"=FALSE, "数值"=w4954, "分辨率"=0.1) -> ("低字节"=w4957:dbl, "高字节1"=w4956:dbl)  [unwired: 2 in, 5 out]
                  }
                  frame Enabled {
                    w4960 = 255 ("高字节1")
                  }
                }
                n1942 = Build Array(w4952, w4953) -> (w4951:i32[])
              }
              frame 1 {
                # "总电压过低"
                n1943 = disable-structure shown="启用" {
                  disable-tunnel: [w4968 w4971] -> w4964
                  disable-tunnel: [w4967 w4971] -> w4963
                  disable-tunnel: w4961 -> [w4966 _]
                  frame Disabled {
